vi "ssh2_exec.vi"() -> ()   [LabVIEW 2017]
doc: "Illustrates how to execute a command on a remote SSH server."
uses:
  libssh2/libssh2_session_handshake_tcp.vi
  libssh2/libssh2_init_default.vi
  libssh2/libssh2_session_init_ex.vi
  <vilib>/Utility/tcp.llb/TCP Get Raw Net Object.vi
  libssh2/libssh2_session_handshake_socket.vi
  libssh2/libssh2_userauth_password_ex.vi
  libssh2/libssh2_channel_open_ex.vi
  libssh2/libssh2_channel_process_startup.vi
  libssh2/libssh2_channel_read_ex.vi
  libssh2/libssh2.lvlib
panel:
  out "standard error":string
  out "exitsignal":string
  out "standard output":string
  out "exit status":i32
  in  "command":string="ping localhost -c 1"
  in  "password":string
  in  "username":string
  out "error out":errorcluster
  in  "hostname":string="localhost"
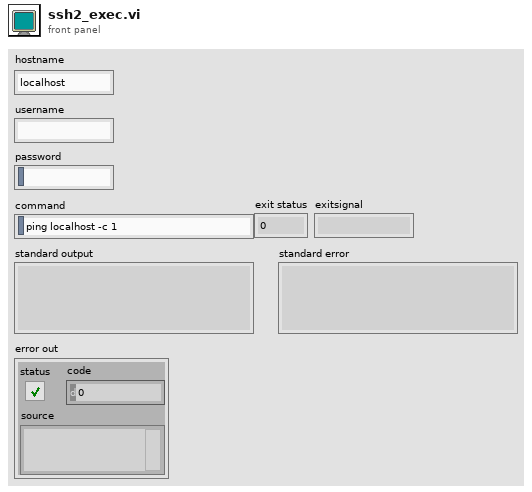
[diagram p1: front panel]
types:
  T1 = typedef "libssh2.lvlib/Session Refnum.ctl" = refnum<k1>
  T2 = typedef "libssh2.lvlib/Channel Refnum.ctl" = refnum<k1>
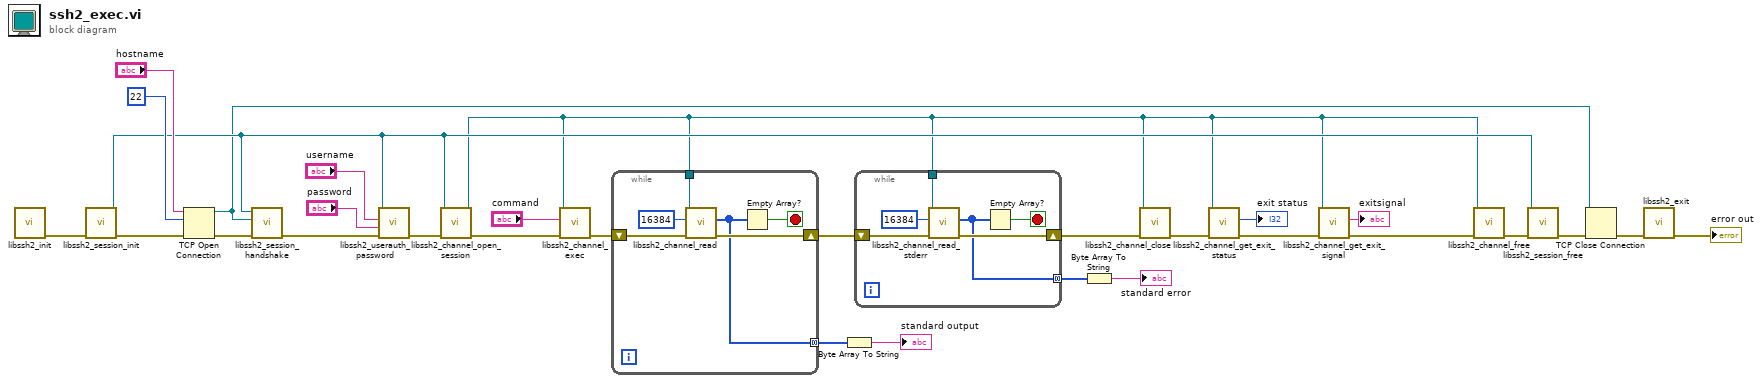
[diagram p0: block diagram]
diagram:
  n1 = call-poly "libssh2_init.vi"() -> ("error out"=w30:errorcluster)  [unwired: 11 in]
  n2 = call "libssh2_session_init.vi"("error in (no error)"=w30) -> ("error out"=w29:errorcluster, "session"=w11:T1)  [unwired: 9 in]
  n3 = TCP Open Connection(address="hostname", remote port or service name=u16 22, error in (no error)=w29) -> (connection ID=w7:refnum<k5>, error out=w8:errorcluster)  [unwired: 2 in]
  n4 = call-poly "libssh2_session_handshake.vi"("error in (no error)"=w8, "tcp connection"=w7, "session"=w11) -> ("error out"=w1:errorcluster)  [unwired: 8 in]
  n5 = call "libssh2_userauth_password.vi"("error in (no error)"=w1, "password"="password", "username"="username", "session"=w11) -> ("error out"=w24:errorcluster)  [unwired: 7 in]
  n6 = call "libssh2_channel_open_session.vi"("error in (no error)"=w24, "session"=w11) -> ("error out"=w21:errorcluster, "channel"=w6:T2)  [unwired: 8 in]
  n7 = call "libssh2_channel_exec.vi"("error in (no error)"=w21, "command"="command", "channel"=w6) -> ("error out"=w20:errorcluster)  [unwired: 8 in]
  n8 = while {
    tunnel: w6 -> [w33]
    tunnel: [w31] -> w13 mode=concatenating
    shift-right: [w35] -> w3
    shift-left: w20 -> [w36]
    stop <- w32 stop-if-true
    n9 = call "libssh2_channel_read.vi"("error in (no error)"=w36, "buffer length"=16384 ("buflen"), "channel"=w33) -> ("error out"=w35:errorcluster, "buffer"=w31:u8[])  [unwired: 7 in]
    n10 = Empty Array?(array=w31) -> (empty?=w32:bool)
  }
  n11 = Byte Array To String(unsigned byte array=w13) -> (string=→"standard output":string)
  n12 = while {
    tunnel: w6 -> [w39]
    tunnel: [w37] -> w4 mode=concatenating
    shift-right: [w41] -> w2
    shift-left: w3 -> [w42]
    stop <- w38 stop-if-true
    n13 = call "libssh2_channel_read_stderr.vi"("error in (no error)"=w42, "buffer length"=16384 ("buflen"), "channel"=w39) -> ("error out"=w41:errorcluster, "buffer"=w37:u8[])  [unwired: 7 in]
    n14 = Empty Array?(array=w37) -> (empty?=w38:bool)
  }
  n15 = Byte Array To String(unsigned byte array=w4) -> (string=→"standard error":string)
  n16 = call "libssh2_channel_close.vi"("error in (no error)"=w2, "channel"=w6) -> ("error out"=w18:errorcluster)  [unwired: 9 in]
  n17 = call "libssh2_channel_get_exit_status.vi"("error in (no error)"=w18, "channel"=w6) -> ("error out"=w17:errorcluster, "exit status"=→"exit status":i32)  [unwired: 8 in]
  n18 = call "libssh2_channel_get_exit_signal.vi"("error in (no error)"=w17, "channel"=w6) -> ("error out"=w16:errorcluster, "exitsignal"=→"exitsignal":string)  [unwired: 6 in, 2 out]
  n19 = call "libssh2_channel_free.vi"("error in (no error)"=w16, "channel"=w6) -> ("error out"=w15:errorcluster)  [unwired: 9 in]
  n20 = call "libssh2_session_free.vi"("error in (no error)"=w15, "session"=w11) -> ("error out"=w28:errorcluster)  [unwired: 9 in]
  n21 = TCP Close Connection(connection ID=w7, error in (no error)=w28) -> (error out=w10:errorcluster)  [unwired: 1 in, 1 out]
  n22 = call "libssh2_exit.vi"("error in (no error)"=w10) -> ("error out"=→"error out":errorcluster)  [unwired: 10 in]
